vi "Receive.vi"(8 "error in (no error)":errorcluster, 11 "Stream in":refnum<class "Stream.lvclass">) -> (0 "error out":errorcluster, 3 "Stream out":refnum<class "Stream.lvclass">)   [LabVIEW 2018, in "Stream.lvclass"]
uses:
  Stream.lvclass
  Stream.lvclass/Stream.ctl
  Comm.lvclass
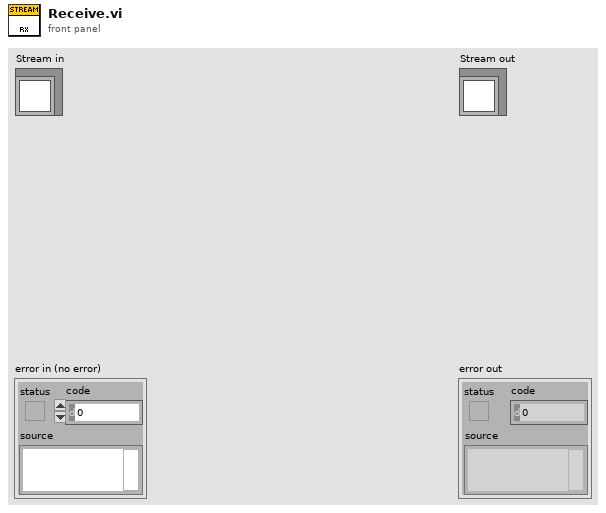
[diagram p1: front panel]
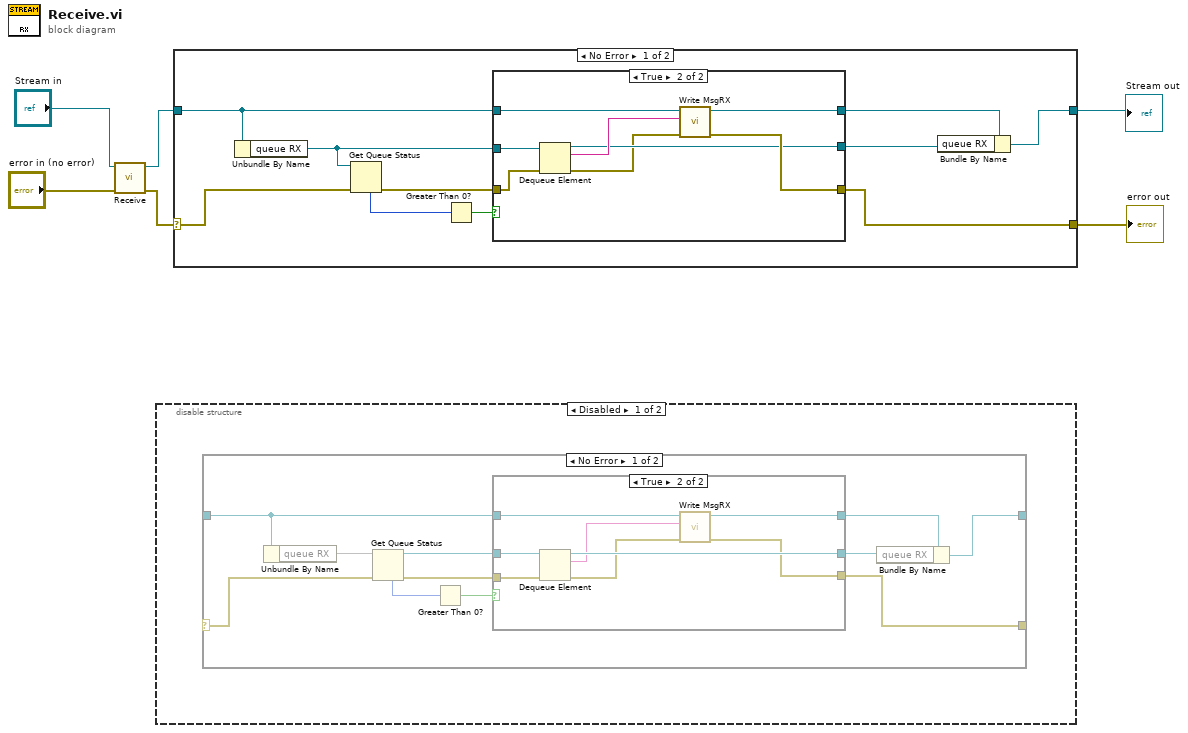
[diagram p0: block diagram]
diagram:
  n1 = call-parent "Receive.vi"("error in (no error)"="error in (no error)", "Comm in"="Stream in") -> ("error out"=w4:errorcluster, "Comm out"=w3:refnum<class "Stream.lvclass">)  [unwired: 8 in]
  n2 = disable-structure shown="Disabled" {
    frame Disabled {
      n3 = case shown="No Error" {
        selector: _ -> [w12 w29]
        tunnel: _ -> [w11 w30]
        tunnel: [w10 w29] -> _
        tunnel: [w8 w30] -> _
        frame No Error {
          n4 = Unbundle By Name(w11) -> ("queue RX"=w17)
          n5 = Get Queue Status(queue=w17, error in (no error)=w12) -> (queue out=w14:refnum<queue>, error out=w13:errorcluster, # elements in queue=w16:i32)  [unwired: 1 in, 5 out]
          n6 = Greater Than 0?(x=w16) -> (x > 0?=w15:bool)
          n7 = case shown="True" w15 {
            tunnel: w14 -> [w19 w28]
            tunnel: w13 -> [w18 w27]
            tunnel: [w19 w26] -> w7
            tunnel: w11 -> [w20 w25]
            tunnel: [w18 w22] -> w10
            tunnel: [w20 w21] -> w9
            frame False {
            }
            frame True {
              n8 = Dequeue Element(queue=w28, error in (no error)=w27) -> (queue out=w26:refnum<queue>, element=w23:string, error out=w24:errorcluster)  [unwired: 1 in, 1 out]
              n9 = call-dynamic "Write MsgRX.vi"("error in (no error)"=w24, "MsgRX"=w23, "Comm in"=w25) -> ("error out"=w22:errorcluster, "Comm out"=w21:refnum<class "Stream.lvclass">)  [unwired: 7 in]
            }
          }
          n10 = Bundle By Name(cluster=w9, "queue RX"=w7) -> (w8:refnum<class "Stream.lvclass">)
        }
        frame Error {
        }
      }
    }
    frame Enabled {
    }
  }
  n11 = case shown="No Error" w4 {
    selector: w4 -> [w31 w52]
    tunnel: w3 -> [w40 w53]
    tunnel: [w39 w52] -> w2
    tunnel: [w36 w53] -> w1
    frame No Error {
      n12 = Unbundle By Name(w40) -> ("queue RX"=w33:refnum<queue>)
      n13 = Get Queue Status(queue=w33, error in (no error)=w31) -> (error out=w32:errorcluster, # elements in queue=w34:i32)  [unwired: 1 in, 6 out]
      n14 = Greater Than 0?(x=w34) -> (x > 0?=w38:bool)
      n15 = case shown="True" w38 {
        tunnel: w33 -> [w42 w48]
        tunnel: w40 -> [w43 w51]
        tunnel: [w41 w50] -> w39
        tunnel: [w43 w49] -> w37
        tunnel: [w42 w46] -> w35
        tunnel: w32 -> [w41 w44]
        frame False {
        }
        frame True {
          n16 = Dequeue Element(queue=w48, error in (no error)=w44) -> (queue out=w46:refnum<queue>, element=w47:string, error out=w45:errorcluster)  [unwired: 1 in, 1 out]
          n17 = call-dynamic "Write MsgRX.vi"("error in (no error)"=w45, "MsgRX"=w47, "Comm in"=w51) -> ("error out"=w50:errorcluster, "Comm out"=w49:refnum<class "Stream.lvclass">)  [unwired: 7 in]
        }
      }
      n18 = Bundle By Name(cluster=w37, "queue RX"=w35) -> (w36:refnum<class "Stream.lvclass">)
    }
    frame Error {
    }
  }
  "error out" <- w2
  "Stream out" <- w1
